vi "exec.vi"(0 "para0":i32, 1 "errmsg":string, 5 "sql":string, 7 "?":i32, 9 "para3":u32, 11 "error in (no error)":errorcluster) -> (3 "errmsg out":string, 4 "para0 out":i32, 6 "function return":i32, 10 "para3 out":u32, 15 "error out":errorcluster)   [LabVIEW 2020, in "sqlite3.lvlib"]
uses:
  sqlite3.lvlib
  errstr.vi
  bin/sqlite3_64.dll
panel:
  # "DO NOT USE"
  # "This uses tricksy callbacks - easier to implement it's component functions in LV"
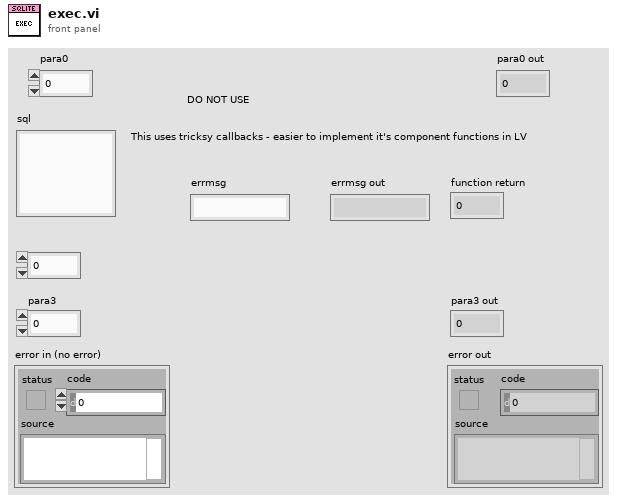
[diagram p1: front panel]
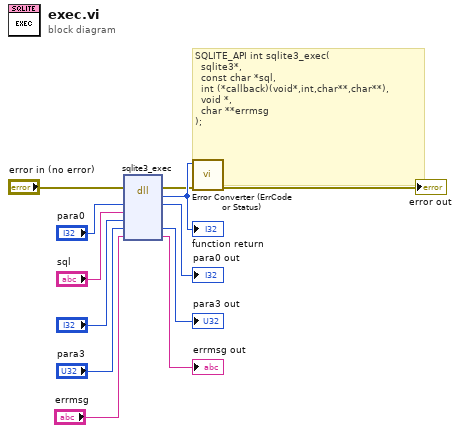
[diagram p0: block diagram]
diagram:
  # "SQLITE_API int sqlite3_exec(\n  sqlite3*,                                  \n  const char *sql,                           \n  int (*callback)(void*,int,char**,char**),  \n  void *,                                    \n  char **errmsg                              \n);"
  n1 = dll-call lib="D:/Project/Labview-Projects/database-configuration/externals/sqlite3/Source/bin/sqlite3_*.*" fn="sqlite3_exec"(error in="error in (no error)", "para0"="para0", "sql"="sql", "arg3"="?", "para3"="para3", "errmsg"="errmsg") -> (error out=w2:errorcluster, "return type"=w12:i32, "para0"=→"para0 out":i32, "para3"=→"para3 out":u32, "errmsg"=→"errmsg out":string)  [unwired: 4 in, 1 out]
  "function return" <- w12
  n2 = call "Error Converter (ErrCode or Status).vi"("error in (no error)"=w2, "error code"=w12) -> ("error out"=→"error out":errorcluster)  [unwired: 9 in]
